vi "OpenPrefDialog.vi"(8 "error in (no error)":errorcluster, 9 "PluginIniFilePath":path, 10 "Class Path":path) -> (0 "error out":errorcluster)   [LabVIEW 2018, in "FgenPlugins.lvlib" / "FgenPluginsBase.lvclass"]
uses:
  FgenPluginsBase.lvclass
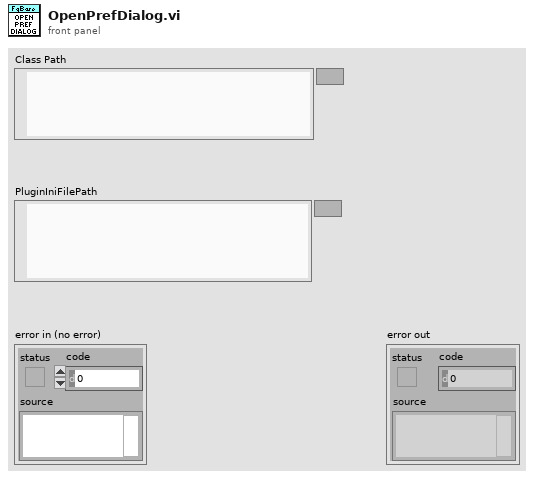
[diagram p1: front panel]
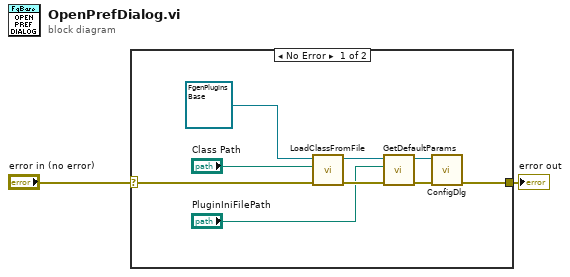
[diagram p0: block diagram]
diagram:
  n1 = case shown="No Error" "error in (no error)" {
    selector: "error in (no error)" -> [w6 w12]
    tunnel: [w7 w12] -> w1
    frame No Error {
      n2 = call-dynamic "LoadClassFromFile.vi"("error in (no error)"=w6, "class path"="Class Path", "reference in"=refnum<class "FgenPluginsBase.lvclass"> refnum ("AcPwrBase in")) -> ("error out"=w11:errorcluster, "reference out"=w10:refnum<class "FgenPluginsBase.lvclass">)  [unwired: 7 in]
      n3 = call-dynamic "GetDefaultParams.vi"("error in (no error)"=w11, "Path"="PluginIniFilePath", "FgenPluginsBase in"=w10) -> ("error out"=w8:errorcluster, "FgenPluginsBase out"=w9:refnum<class "FgenPluginsBase.lvclass">)  [unwired: 7 in]
      n4 = call-dynamic "ConfigDlg.vi"("error in (no error)"=w8, "FgenPluginsBase in"=w9) -> ("error out"=w7:errorcluster)  [unwired: 7 in, 2 out]
    }
    frame Error {
    }
  }
  "error out" <- w1
